vi "SQL_Table_Test_Select.vi"() -> (7 "error out":errorcluster, 10 "表格控件":string[][](table))   [LabVIEW 2014]
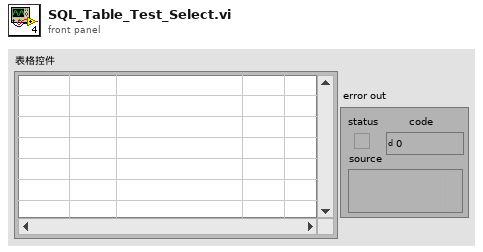
[diagram p1: front panel]
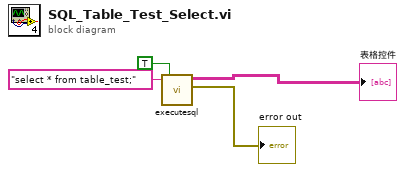
[diagram p0: block diagram]
diagram:
  n1 = call "executesql.vi"("Return Data (T)"=TRUE, "Command Text"="select * from table_test;") -> ("error out"=→"error out":errorcluster, "Data"=→"表格控件":string[][])  [unwired: 5 in]
